vi "ExpBtn.vi"() -> ()   [LabVIEW 2009]
panel:
  in  "stop":bool
  in  "Boton 2":bool
  in  "Boton 1":bool
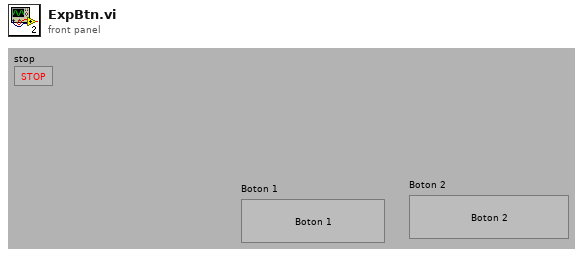
[diagram p1: front panel]
types:
  T1 = enum8{"Enabled", "Disabled", "Disabled and Grayed Out"}
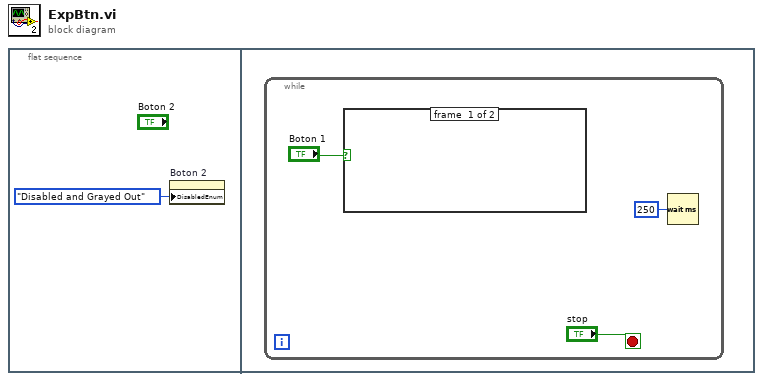
[diagram p0: block diagram]
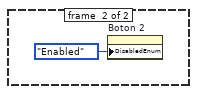
[diagram p2: hidden frame]
diagram:
  n1 = flat-sequence {
    frame #0 {
      n2 = property on="Boton 2" class="Bool"("DisabledEnum"=T1."Disabled and Grayed Out" ("Désactivé")) -> ()  [unwired: 2 in, 2 out]
    }
    frame #1 {
      n3 = while {
        stop <- "stop" stop-if-true
        n4 = case shown="Vrai" "Boton 1" {
          frame #0 {
          }
          frame #1 {
            n5 = property on="Boton 2" class="Bool"("DisabledEnum"=T1."Enabled" ("Désactivé")) -> ()  [unwired: 2 in, 2 out]
          }
        }
        n6 = Wait (ms)(milliseconds to wait=u32 250 ("attente (ms)")) -> ()  [unwired: 1 out]
      }
    }
  }
